vi "SinCos4.vi"() -> (8 "SinCos4":refnum<class "SinCos4.lvclass">)   [LabVIEW 2017, in "SinCos4.lvclass"]
uses:
  SinCos4.lvclass
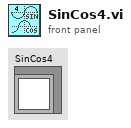
[diagram p1: front panel]
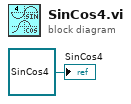
[diagram p0: block diagram]
diagram:
  "SinCos4" <- refnum<class "SinCos4.lvclass"> refnum ("SinCos4.lvclass")
